vi "Build.vi"() -> ()   [LabVIEW 2011]
uses:
  <vilib>/JKI/VIPM API/VIPM API_vipm_api.lvlib
panel:
  out "error out":errorcluster
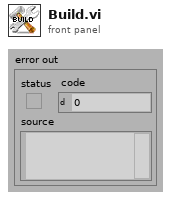
[diagram p1: front panel]
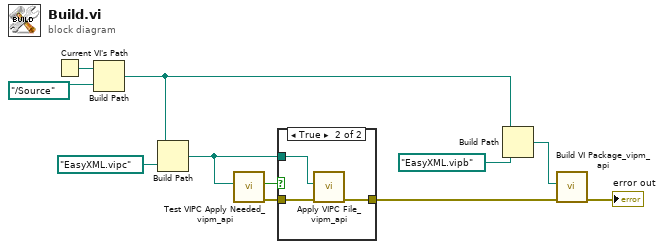
[diagram p0: block diagram]
diagram:
  n1 = Current VI's Path() -> (path=w11:path)
  n2 = Build Path(base path=w11, name or relative path=path "../Source" ("Path to VIPB File")) -> (appended path=w6:path)
  n3 = Build Path(base path=w6, name or relative path=path "EasyXML.vipc" ("Path to VIPB File")) -> (appended path=w4:path)
  n4 = call <vilib>:"Test VIPC Apply Needed_vipm_api.vi"("VIPC File Path"=w4) -> ("error out"=w3:errorcluster, "Need to Apply?"=w5:bool)  [unwired: 9 in]
  n5 = case shown="True" w5 {
    tunnel: w4 -> [_ w15]
    tunnel: w3 -> [w12 w14]
    tunnel: [w12 w13] -> w2
    frame False {
    }
    frame True {
      n6 = call <vilib>:"Apply VIPC File_vipm_api.vi"("error in (no error)"=w14, "VIPC File"=w15) -> ("error out"=w13:errorcluster)  [unwired: 9 in]
    }
  }
  n7 = Build Path(base path=w6, name or relative path=path "EasyXML.vipb" ("Path to VIPB File")) -> (appended path=w1:path)
  n8 = call <vilib>:"Build VI Package_vipm_api.vi"("error in (no error)"=w2, "Path to VIPB File"=w1) -> ("error out"=→"error out":errorcluster)  [unwired: 8 in, 1 out]
